vi "get_reference_by_label.vi"(8 "error in":errorcluster, 11 "Label":string) -> (0 "error out":errorcluster, 2 "Encontrado?":bool, 3 "Ctl Refnum":refnum<vi>)   [LabVIEW 2018]
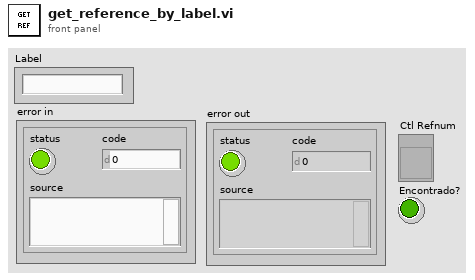
[diagram p1: front panel]
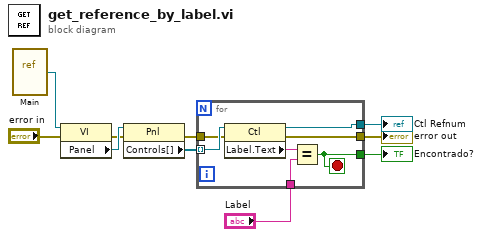
[diagram p0: block diagram]
diagram:
  n1 = vi-ref "Main.vi"() -> (w10:refnum<vi>)
  n2 = property class="VI"(reference=w10, error in="error in") -> (error out=w4:errorcluster, "Panel"=w9:refnum<vi>)  [unwired: 1 out]
  n3 = property class="Pnl"(reference=w9, error in=w4) -> (error out=w3:errorcluster, "Controls[]"=w8:refnum<vi>[])  [unwired: 1 out]
  n4 = for {
    tunnel: w8 -> [w17] mode=indexing
    tunnel: "Label" -> [w15]
    tunnel: [w14] -> w6
    tunnel: w3 -> [w13]
    tunnel: [w12] -> w2
    tunnel: [w11] -> w1
    stop <- w11 stop-if-true
    n5 = property class="Ctl"(reference=w17, error in=w13) -> (reference out=w14:refnum<vi>, error out=w12:errorcluster, "Label.Text"=w16:string)
    n6 = Equal?(x=w16, y=w15) -> (x = y?=w11:bool)
  }
  "Ctl Refnum" <- w6
  "error out" <- w2
  "Encontrado?" <- w1
